vi "Lockin.Mixer.vi"(8 "error in (no error)":errorcluster, 11 "DSP in":refnum<class "DSP.lvclass">) -> (0 "error out":errorcluster, 3 "DSP out":refnum<class "DSP.lvclass">)   [LabVIEW 2019, in "DSP.lvclass"]
uses:
  DSP.lvclass
  DSP.lvclass/DSP.ctl
  Waveform.Attributes/Waveform.Attributes.lvlib
panel:
  out "Waveforms out":T1
  out "Waveforms in":T1
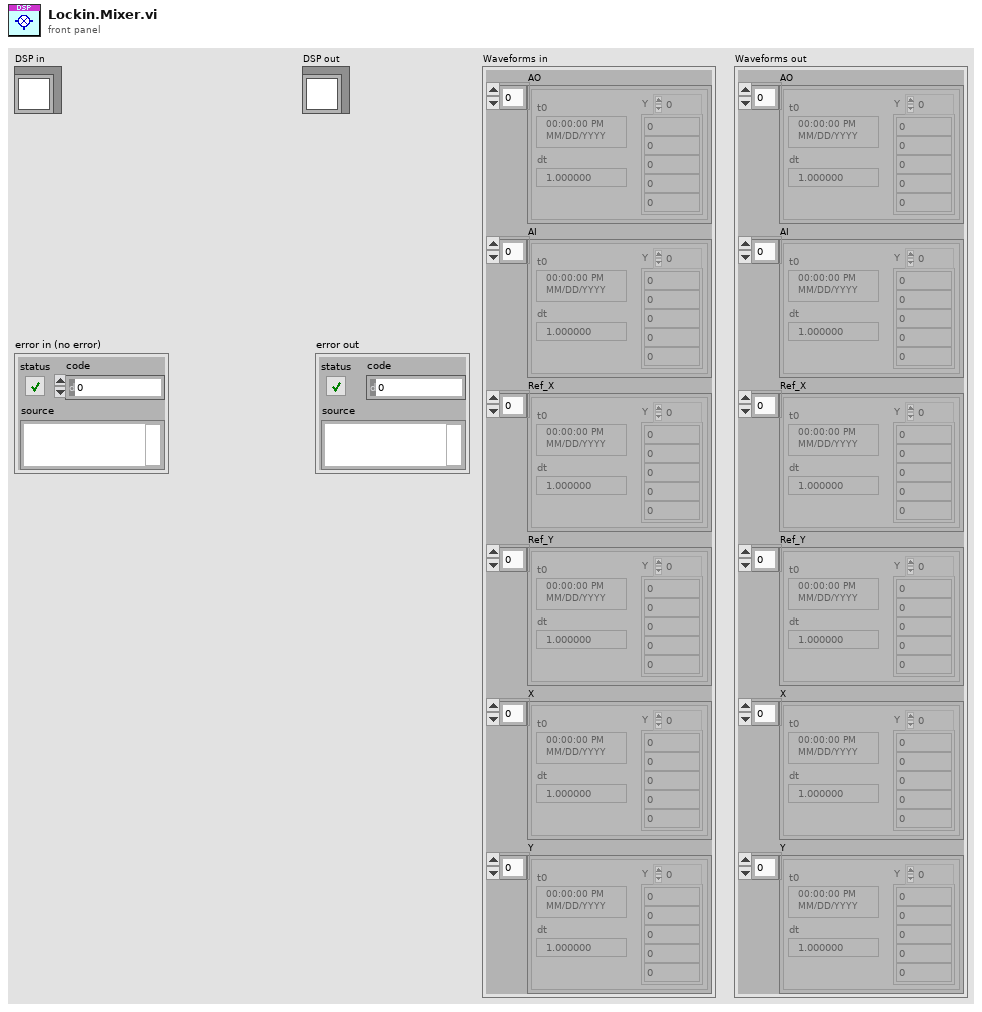
[diagram p1: front panel]
types:
  T1 = cluster{"AO":waveform(dbl)[], "AI":waveform(dbl)[], "Ref_X":waveform(dbl)[], "Ref_Y":waveform(dbl)[], "X":waveform(dbl)[], "Y":waveform(dbl)[]}
  T2 = typedef "DSP.lvclass/AI.Channel--Cluster--Array.ctl" = T3[]
  T3 = typedef "DSP.lvclass/AI.Channel--Cluster.ctl" = cluster{"Enable?":bool, "Channel":i32, "References":i32[], "reference index":i32}
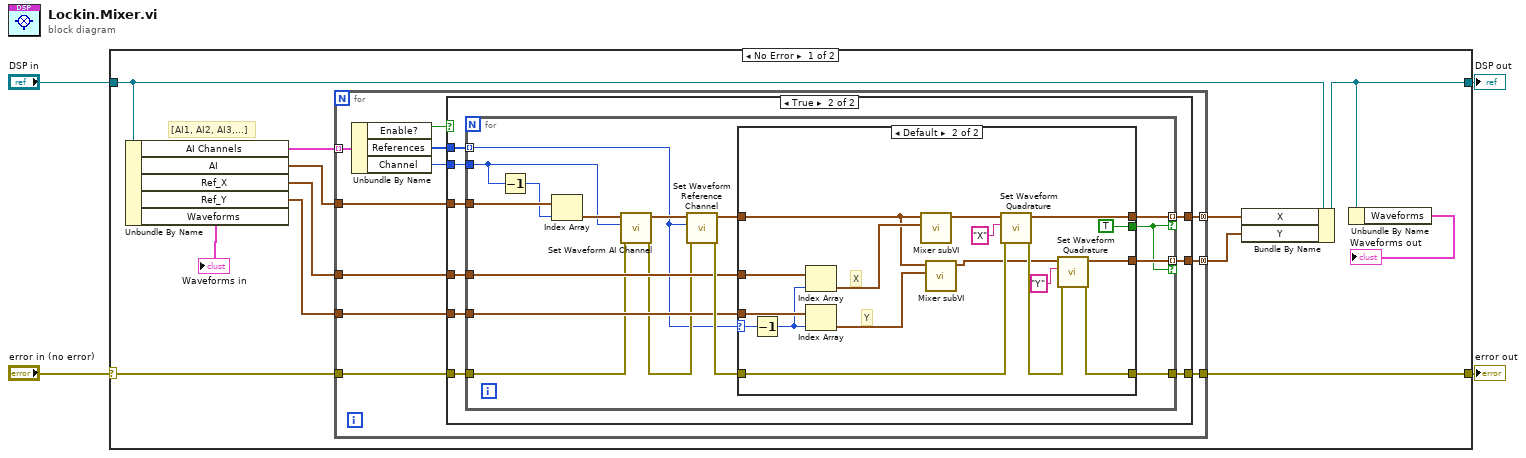
[diagram p0: block diagram]
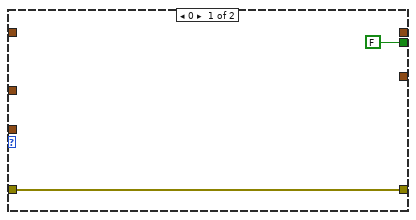
[diagram p3: hidden frame]
diagram:
  n1 = case shown="No Error" "error in (no error)" {
    selector: "error in (no error)" -> [w14 w74]
    tunnel: [w16 w74] -> w4
    tunnel: "DSP in" -> [w15 w73]
    tunnel: [w6 w73] -> w2
    frame No Error {
      # "[AI1, AI2, AI3,...]"
      n2 = Unbundle By Name(w15) -> ("AI Channels"=w9:T2, "AI"=w13:waveform(dbl)[], "Ref_X"=w12:waveform(dbl)[], "Ref_Y"=w11:waveform(dbl)[], "Waveforms"=→"Waveforms in":T1)
      n3 = for {
        tunnel: [w26] -> w8 mode=concatenating
        tunnel: w13 -> [w22]
        tunnel: w9 -> [w20] mode=indexing
        tunnel: w12 -> [w25]
        tunnel: w11 -> [w24]
        tunnel: [w23] -> w10 mode=concatenating
        tunnel: w14 -> [w21]
        tunnel: [w27] -> w16
        n4 = Unbundle By Name(w20) -> ("Enable?"=w17:bool, "References"=w19:i32[], "Channel"=w18:i32)
        n5 = case shown="True" w17 {
          tunnel: [w28 w37] -> w27
          tunnel: [_ w36] -> w26
          tunnel: w25 -> [_ w35]
          tunnel: w24 -> [_ w34]
          tunnel: [_ w33] -> w23
          tunnel: w22 -> [_ w32]
          tunnel: w21 -> [w28 w31]
          tunnel: w19 -> [_ w30]
          tunnel: w18 -> [_ w29]
          frame False {
          }
          frame True {
            n6 = for {
              tunnel: [w50] -> w36 mode=indexing if=w46
              tunnel: w35 -> [w49]
              tunnel: w34 -> [w48]
              tunnel: [w47] -> w33 mode=indexing if=w46
              tunnel: w32 -> [w45]
              tunnel: w31 -> [w41]
              tunnel: [w53] -> w37
              tunnel: w30 -> [w40] mode=indexing
              tunnel: w29 -> [w38]
              n7 = Decrement(x=w38) -> (x-1=w43:i32)
              n8 = Index Array(array=w45, index=w43) -> (element=w39:waveform(dbl))
              n9 = call "Set Waveform AI Channel.vi"("error in (no error)"=w41, "AI Channel"=w38, "Waveform in"=w39) -> ("error out"=w42:errorcluster, "Waveform out"=w44:waveform(dbl))  [unwired: 7 in]
              n10 = call "Set Waveform Reference Channel.vi"("error in (no error)"=w42, "Reference Ch"=w40, "Waveform in"=w44) -> ("error out"=w51:errorcluster, "Waveform out"=w52:waveform(dbl))  [unwired: 7 in]
              n11 = case shown="Default" w40 {
                selector: w40 -> [_ w69]
                tunnel: [w55 w67] -> w53
                tunnel: w52 -> [_ w58]
                tunnel: w51 -> [w55 w61]
                tunnel: [_ w62] -> w50
                tunnel: [FALSE TRUE] -> w46
                tunnel: w49 -> [_ w71]
                tunnel: w48 -> [_ w70]
                tunnel: [_ w60] -> w47
                frame 0 {
                }
                frame Default {
                  # "Y"
                  # "X"
                  n12 = Decrement(x=w69) -> (x-1=w64:i32)
                  n13 = Index Array(array=w71, index=w64) -> (element=w59:waveform(dbl))
                  n14 = Index Array(array=w70, index=w64) -> (element=w56:waveform(dbl))
                  n15 = call "Mixer subVI.vi"("Reference in"=w59, "Signal in"=w58) -> ("Signal*Reference out"=w63:waveform(dbl))  [unwired: 9 in]
                  n16 = call "Mixer subVI.vi"("Reference in"=w56, "Signal in"=w58) -> ("Signal*Reference out"=w57:waveform(dbl))  [unwired: 9 in]
                  n17 = call "Set Waveform Quadrature.vi"("error in (no error)"=w61, "Quadratude"="X", "Waveform in"=w63) -> ("error out"=w68:errorcluster, "Waveform out"=w62:waveform(dbl))  [unwired: 7 in]
                  n18 = call "Set Waveform Quadrature.vi"("error in (no error)"=w68, "Quadratude"="Y", "Waveform in"=w57) -> ("error out"=w67:errorcluster, "Waveform out"=w60:waveform(dbl))  [unwired: 7 in]
                }
              }
            }
          }
        }
      }
      n19 = Bundle By Name(cluster=w15, "X"=w8, "Y"=w10) -> (w6:refnum<class "DSP.lvclass">)
      n20 = Unbundle By Name(w6) -> ("Waveforms"=→"Waveforms out":T1)
    }
    frame Error {
    }
  }
  "error out" <- w4
  "DSP out" <- w2
